vi "Updater Event Log.vi"(8 "error in (no error)":errorcluster, 11 "Log Entry":string) -> (0 "error out":errorcluster)   [LabVIEW 2011]
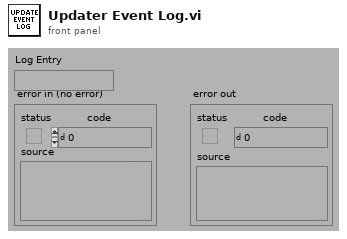
[diagram p1: front panel]
types:
  T1 = enum16{"open", "replace", "create", "open or create", "replace or create", "replace or create with confirmation"}
  T2 = enum32{"invalid app kind", "Development System", "Run Time System", "Student Edition", "Embedded LabVIEW", "Evaluation", "Custom"}
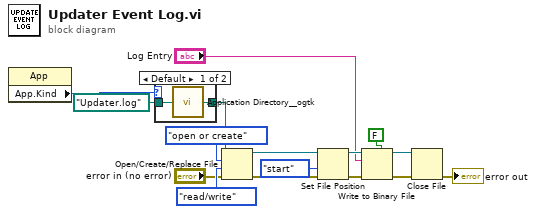
[diagram p0: block diagram]
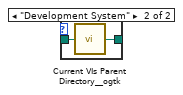
[diagram p2: hidden frame]
diagram:
  n1 = property class="App"() -> ("App.Kind"=w16:T2)  [unwired: 2 in, 2 out]
  n2 = case shown="Default" w16 {
    tunnel: [w18 w20] -> w4
    tunnel: path "Updater.log" -> [w17 w19]
    frame Default {
      n3 = call "Application Directory__ogtk.vi"("Relative path (.)"=w17) -> ("Application Directory (+ Relative)"=w18:path)
    }
    frame "Development System" {
      n4 = call "Current VIs Parent Directory__ogtk.vi"("Relative path (.)"=w19) -> ("Parent Directory (+ Relative)"=w20:path)  [unwired: 4 out]
    }
  }
  n5 = Open/Create/Replace File(file path (use dialog)=w4, error in="error in (no error)", operation (0:open)=T1."open or create", access (0:read/write)=enum16{"read/write", "read-only", "write-only"}."read/write") -> (refnum out=w7:refnum<file>, error out=w6:errorcluster)  [unwired: 3 out]
  n6 = Set File Position(refnum=w7, from (0:start)=enum16{"start", "end", "current"}."start", error in=w6) -> (refnum out=w10:refnum<file>, error out=w11:errorcluster)  [unwired: 1 out]
  n7 = Write to Binary File(file (use dialog)=w10, data="Log Entry", error in=w11, 5:FALSE) -> (refnum out=w14:refnum<file>, error out=w13:errorcluster)  [unwired: 3 out]
  n8 = Close File(refnum=w14, error in=w13) -> (error out=→"error out":errorcluster)  [unwired: 1 out]
